vi "Jog Mode.vi"(6 "Speed":i32, 8 "error in (no error)":errorcluster, 9 "uStep":i32, 10 "wfmStep":i32, 11 "Inst.MOTOR in":refnum<class "Inst.MOTOR.lvclass">) -> (0 "error out":errorcluster, 3 "Inst.MOTOR out":refnum<class "Inst.MOTOR.lvclass">)   [LabVIEW 2019, in "Inst.MOTOR.lvclass"]
uses:
  Inst.MOTOR.lvclass
panel:
  out "read buffer":string
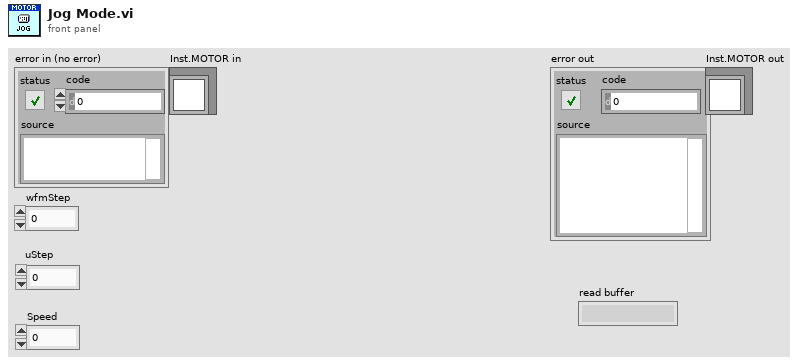
[diagram p1: front panel]
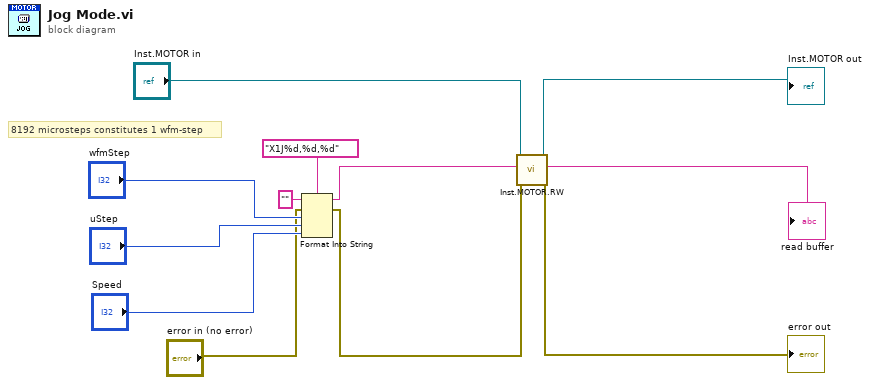
[diagram p0: block diagram]
diagram:
  # "8192 microsteps constitutes 1 wfm-step"
  n1 = Format Into String(format string="X1J%d,%d,%d", initial string="", error in="error in (no error)", "wfmStep", "uStep", "Speed") -> (resulting string=w7:string, error out=w2:errorcluster)
  n2 = call "Inst.MOTOR.RW.vi"("error in (no error)"=w2, "Data in"=w7, "Inst.MOTOR in"="Inst.MOTOR in") -> ("error out"=→"error out":errorcluster, "read buffer"=→"read buffer":string, "Inst.MOTOR out"=→"Inst.MOTOR out":refnum<class "Inst.MOTOR.lvclass">)  [unwired: 6 in]
